vi "QuickProfile_V2.vi"(7 "Image IN":sgl[][](array[numeric]), 11 "Pixel Size (nm)":dbl, 13 "Test Image":bool) -> ()   [LabVIEW 2012]
uses:
  <vilib>/Utility/file.llb/Write To Spreadsheet File (DBL).vi
panel:
  in  "Open Image":bool
  in  "Save ROI":bool
  in  "Power (%)":dbl
  in  "Delay (ps)":dbl
  out "Lorentzian Fit Width (nm)":dbl
  out "Gaussian Fit Width Y (nm)":dbl
  out "Gaussian Fit Width X (nm)":dbl
  in  "Auto Save":bool
  in  "Save Data":bool
  in  "Save File":path
  out "Constant Y Slice":cluster{"X Values":dbl[], sgl[]}[](graph)
  out "Constant X Slice":cluster{"X Values":dbl[], sgl[]}[](graph)
  in  "Fit ROI":bool
  out "Gaussian Fit":dbl[][](graph)
  out "Lorentzian Fit":dbl[][](graph)
  out "Current ROI":sgl[][](graph)
  in  "Region Size (px)":dbl=60.0
  in  "Quit":bool
  out "Image Display":sgl[][](graph)
  # "Constant Y"
  # "Constant X"
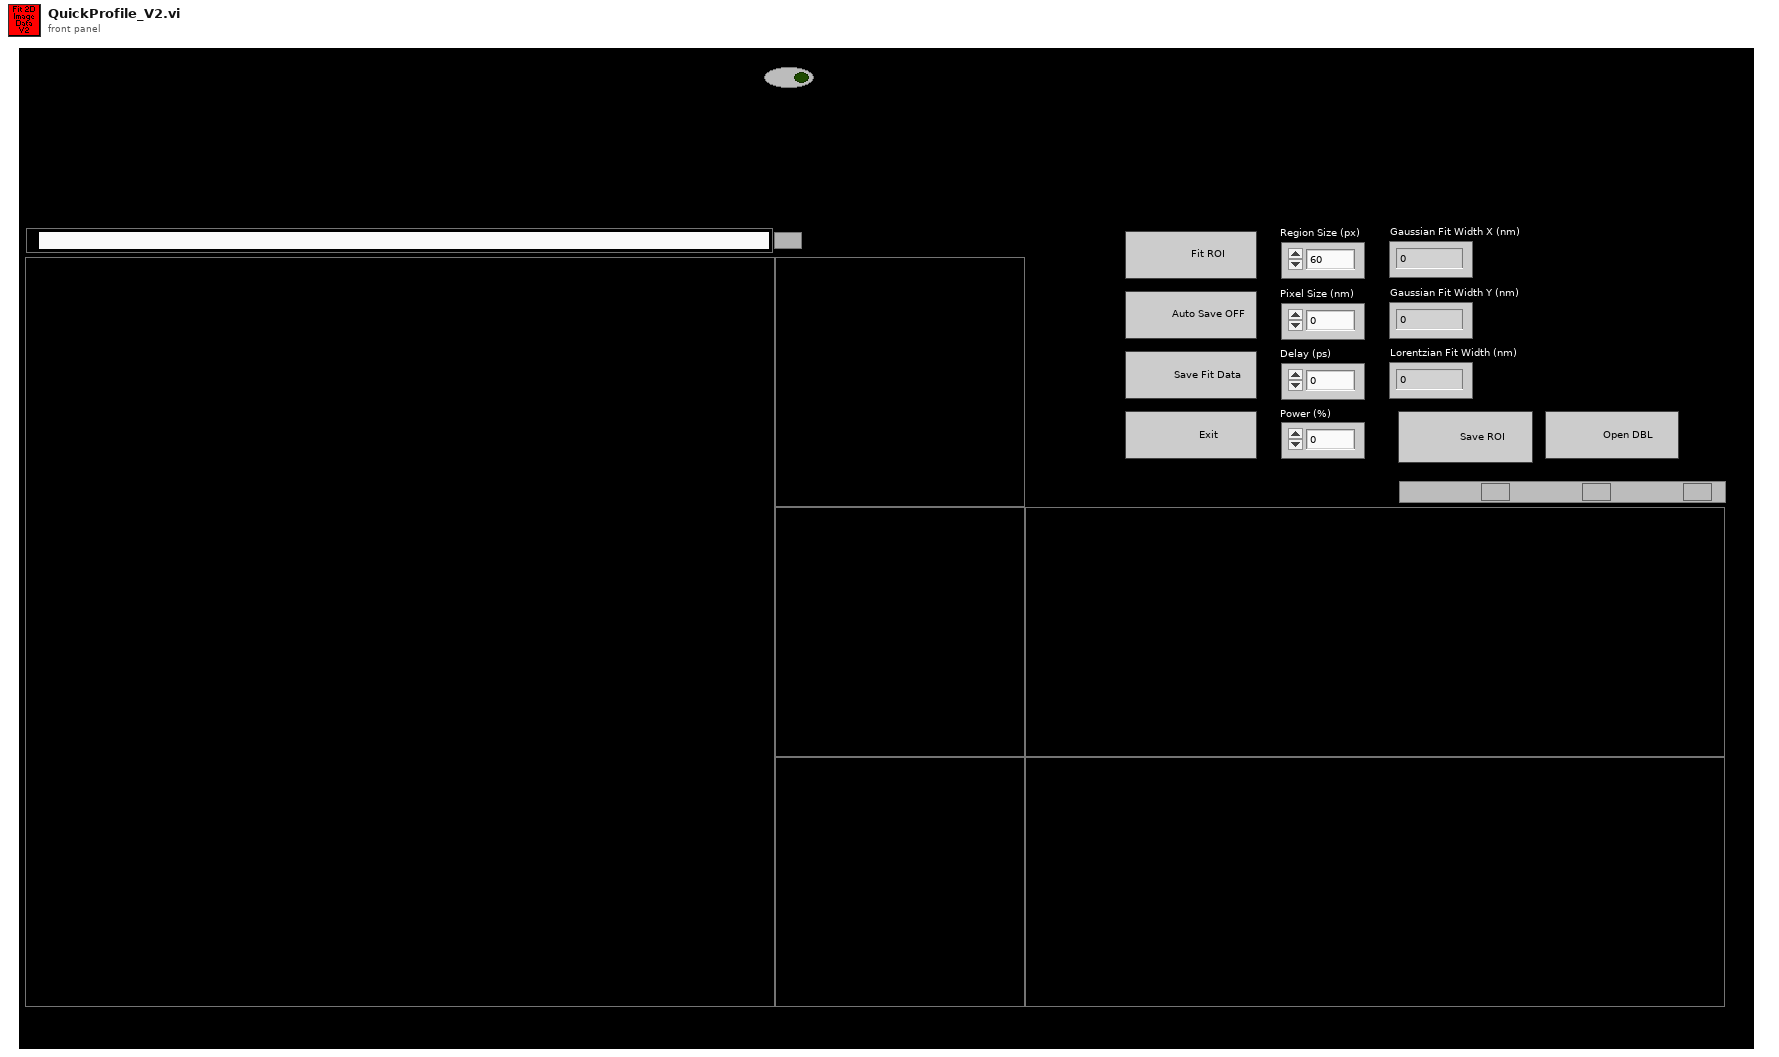
[diagram p1: front panel]
types:
  T1 = enum16{"open", "replace", "create", "open or create", "replace or create", "replace or create with confirmation"}
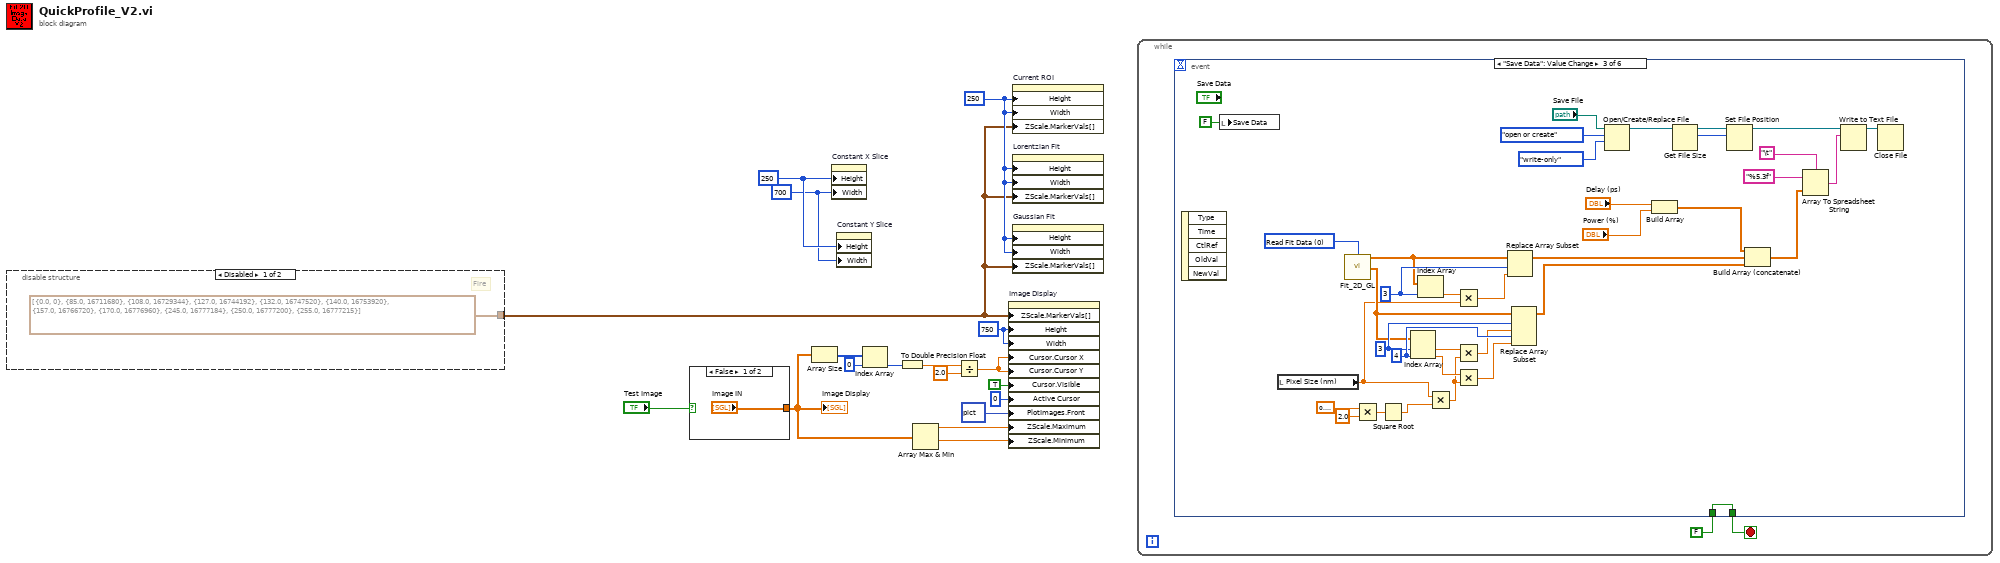
[diagram p0: block diagram]
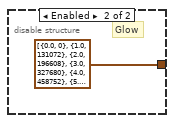
[diagram p2: hidden frame]
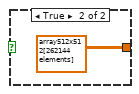
[diagram p3: hidden frame]
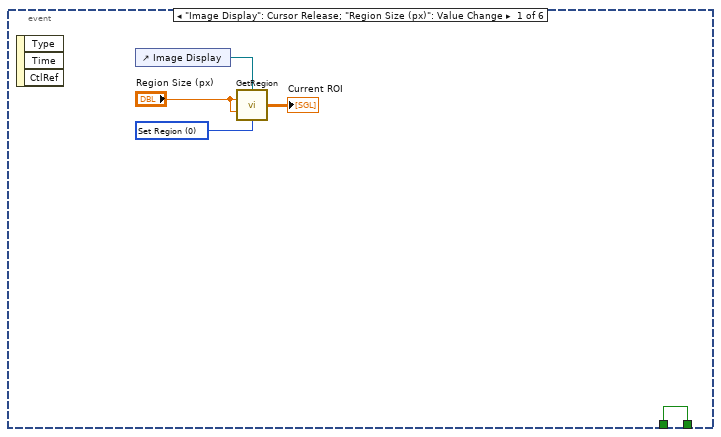
[diagram p4: hidden frame]
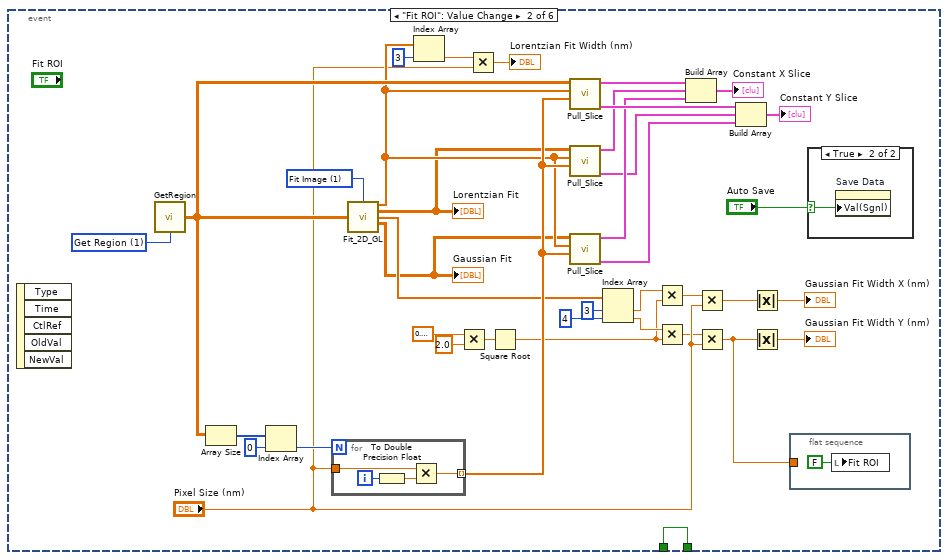
[diagram p5: hidden frame]
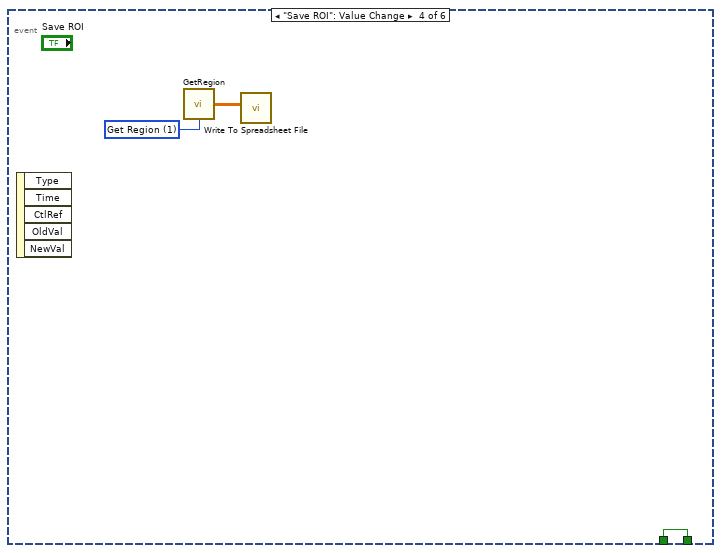
[diagram p7: hidden frame]
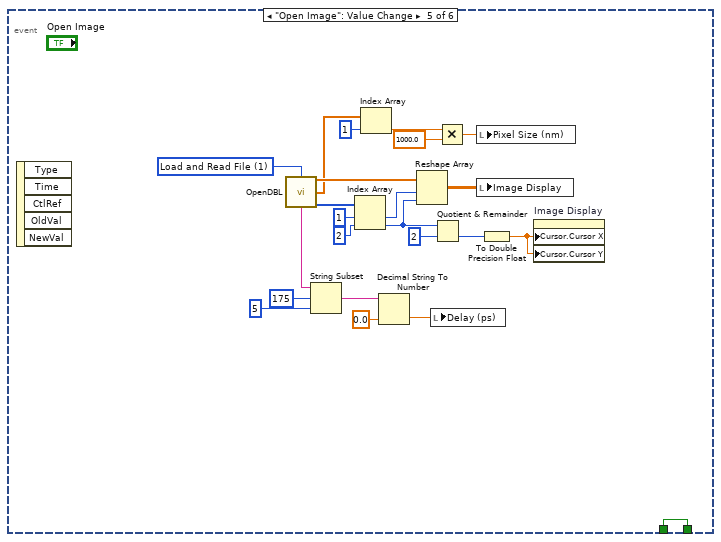
[diagram p8: hidden frame]
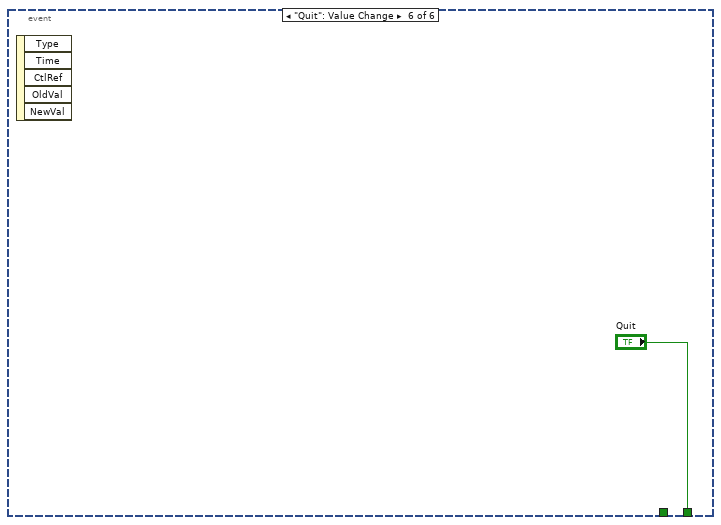
[diagram p9: hidden frame]
diagram:
  w11 = u32 700 ("Plot Area:Size:Width")
  w12 = u32 250 ("Plot Area:Size:Height")
  w14 = u32 250 ("Plot Area:Size:Height")
  w18 = u32 750 ("Plot Area:Size:Height")
  n1 = disable-structure shown="Disabled" {
    disable-tunnel: [cluster{dbl, u32}[] [{0.0, 0}, {85.0, 16711680}, {108.0, 16729344}, {127.0, 16744192}, {132.0, 16747520}, {140.0, 16753920}, {157.0, 16766720}, {170.0, 16776960}, {245.0, 16777184}, {250.0, 16777200}, {255.0, 16777215}] ("Z Scale.Marker Values[]") cluster{dbl, u32}[] [{0.0, 0}, {1.0, 131072}, {2.0, 196608}, {3.0, 327680}, {4.0, 458752}, {5.0, 589824}, {6.0, 720896}, {7.0, 851971}, {8.0, 983043}, {9.0, 1114115}, {10.0, 1245187}, {11.0, 1376259}, {12.0, 1507331}, {13.0, 1638403}, {14.0, 1769475}, {15.0, 1769479}, {16.0, 2031623}, {17.0, 2162695}, {18.0, 2293767}, {19.0, 2424839}, {20.0, 2555911}, {21.0, 2686983}, {22.0, 2818055}, {23.0, 2949127}, {24.0, 3080203}, {25.0, 3211275}, {26.0, 3342347}, {27.0, 3473419}, {28.0, 3604491}, {29.0, 3735563}, {30.0, 3866635}, {31.0, 3867403}, {32.0, 4129547}, {33.0, 4260619}, {34.0, 4391691}, {35.0, 4522763}, {36.0, 4653839}, {37.0, 4784911}, {38.0, 4915983}, {39.0, 5178127}, {40.0, 5309199}, {41.0, 5440271}, {42.0, 5571343}, {43.0, 5702415}, {44.0, 5703439}, {45.0, 5965583}, {46.0, 6096655}, {47.0, 6227727}, {48.0, 6358799}, {49.0, 6489871}, {50.0, 6620943}, {51.0, 6752015}, {52.0, 6883087}, {53.0, 7015183}, {54.0, 7146255}, {55.0, 7277327}, {56.0, 7408399}, {57.0, 7539471}, {58.0, 7670543}, {59.0, 7801615}, {60.0, 8063759}, {61.0, 8194831}, {62.0, 8326927}, {63.0, 8457999}, {64.0, 8589075}, {65.0, 8720147}, {66.0, 8851219}, {67.0, 8982291}, {68.0, 9113363}, {69.0, 9114387}, {70.0, 9376531}, {71.0, 9507603}, {72.0, 9638675}, {73.0, 9769747}, {74.0, 9901843}, {75.0, 10032915}, {76.0, 10163987}, {77.0, 10229523}, {78.0, 10295059}, {79.0, 10427155}, {80.0, 10558227}, {81.0, 10689299}, {82.0, 10820371}, {83.0, 10886931}, {84.0, 10952467}, {85.0, 11083539}, {86.0, 11214611}, {87.0, 11215635}, {88.0, 11477779}, {89.0, 11543315}, {90.0, 11608851}, {91.0, 11740947}, {92.0, 11806483}, {93.0, 11872019}, {94.0, 12004115}, {95.0, 12135187}, {96.0, 12266259}, {97.0, 12267283}, {98.0, 12398355}, {99.0, 12529427}, {100.0, 12530451}, {101.0, 12595987}, {102.0, 12530451}, {103.0, 12793619}, {104.0, 12794131}, {105.0, 12794643}, {106.0, 13056787}, {107.0, 13057299}, {108.0, 13057811}, {109.0, 13188883}, {110.0, 13320979}, {111.0, 13386515}, {112.0, 13452563}, {113.0, 13584147}, {114.0, 13584659}, {115.0, 13585171}, {116.0, 13585683}, {117.0, 13717267}, {118.0, 13848339}, {119.0, 13849363}, {120.0, 13849875}, {121.0, 13850387}, {122.0, 13981459}, {123.0, 14113555}, {124.0, 14114067}, {125.0, 14114579}, {126.0, 14115091}, {127.0, 14246675}, {128.0, 14377747}, {129.0, 14378771}, {130.0, 14379283}, {131.0, 14379539}, {132.0, 14379795}, {133.0, 14380819}, {134.0, 14511891}, {135.0, 14643987}, {136.0, 14644503}, {137.0, 14645015}, {138.0, 14645527}, {139.0, 14646039}, {140.0, 14646551}, {141.0, 14778135}, {142.0, 14909207}, {143.0, 14910231}, {144.0, 14910747}, {145.0, 14911259}, {146.0, 14911771}, {147.0, 14912283}, {148.0, 14912797}, {149.0, 15044383}, {150.0, 15175455}, {151.0, 15175967}, {152.0, 15176479}, {153.0, 15176991}, {154.0, 15177507}, {155.0, 15178019}, {156.0, 15178531}, {157.0, 15310115}, {158.0, 15441701}, {159.0, 15441959}, {160.0, 15442215}, {161.0, 15442727}, {162.0, 15443243}, {163.0, 15443755}, {164.0, 15444269}, {165.0, 15444783}, {166.0, 15444783}, {167.0, 15576367}, {168.0, 15707953}, {169.0, 15708467}, {170.0, 15708979}, {171.0, 15708981}, {172.0, 15708983}, {173.0, 15710011}, {174.0, 15710523}, {175.0, 15711037}, {176.0, 15711039}, {177.0, 15711553}, {178.0, 15843139}, {179.0, 15974213}, {180.0, 15974215}, {181.0, 15974217}, {182.0, 15974219}, {183.0, 15975755}, {184.0, 15976271}, {185.0, 15976785}, {186.0, 15977299}, {187.0, 15977301}, {188.0, 15977815}, {189.0, 15978327}, {190.0, 15978331}, {191.0, 16109917}, {192.0, 16241503}, {193.0, 16241505}, {194.0, 16242019}, {195.0, 16242535}, {196.0, 16242537}, {197.0, 16242539}, {198.0, 16243563}, {199.0, 16243567}, {200.0, 16244081}, {201.0, 16244595}, {202.0, 16244599}, {203.0, 16244601}, {204.0, 16244603}, {205.0, 16245627}, {206.0, 16245631}, {207.0, 16245633}, {208.0, 16246147}, {209.0, 16246663}, {210.0, 16377735}, {211.0, 16508811}, {212.0, 16508815}, {213.0, 16509839}, {214.0, 16509843}, {215.0, 16509845}, {216.0, 16509847}, {217.0, 16510361}, {218.0, 16510875}, {219.0, 16510879}, {220.0, 16510881}, {221.0, 16510883}, {222.0, 16511399}, {223.0, 16511911}, {224.0, 16511915}, {225.0, 16511917}, {226.0, 16511919}, {227.0, 16511923}, {228.0, 16512437}, {229.0, 16512951}, {230.0, 16512955}, {231.0, 16512957}, {232.0, 16512959}, {233.0, 16512961}, {234.0, 16512963}, {235.0, 16512967}, {236.0, 16513481}, {237.0, 16513995}, {238.0, 16513999}, {239.0, 16514001}, {240.0, 16514003}, {241.0, 16514005}, {242.0, 16514007}, {243.0, 16514011}, {244.0, 16514013}, {245.0, 16514015}, {246.0, 16514019}, {247.0, 16514021}, {248.0, 16514023}, {249.0, 16514027}, {250.0, 16514029}, {251.0, 16514031}, {252.0, 16514035}, {253.0, 16514037}, {254.0, 16514039}, {255.0, 16514043}] ("Z Scale.Marker Values[]")] -> w13
    frame Disabled {
      # "Fire"
    }
    frame Enabled {
      # "Glow"
    }
  }
  n2 = case shown="False" "Test Image" {
    tunnel: ["Image IN" sgl[][] array512x512[262144 elements] ("Im Prev")] -> w7
    frame False {
    }
    frame True {
    }
  }
  "Image Display" <- w7
  n3 = Array Size(array=w7) -> (size(s)=w6:i32[])
  n4 = property on="Constant X Slice" class="XYGraph (strict)"("Height"=w12, "Width"=w11) -> ()  [unwired: 2 in, 2 out]
  n5 = property on="Constant Y Slice" class="XYGraph (strict)"("Height"=w12, "Width"=w11) -> ()  [unwired: 2 in, 2 out]
  n6 = Index Array(array=w6, index=0) -> (element=w4:i32)
  n7 = To Double Precision Float(number=w4) -> (double precision float=w2:dbl)
  n8 = Array Max & Min(array=w7) -> (max value=w10:sgl, min value=w9:sgl)  [unwired: 2 out]
  n9 = Divide(x=w2, y=2.0) -> (x/y=w1:dbl)
  n10 = property on="Image Display" class="IntGraph (strict)"("ZScale.MarkerVals[]"=w13, "Height"=w18, "Width"=w18, "Cursor.Cursor X"=w1, "Cursor.Cursor Y"=w1, "Cursor.Visible"=TRUE, "Active Cursor"=u32 0, "PlotImages.Front"=picture data[5B] ("Plot Images:Front"), "ZScale.Maximum"=w10, "ZScale.Minimum"=w9) -> ()  [unwired: 2 in, 2 out]
  n11 = property on="Current ROI" class="IntGraph (strict)"("Height"=w14, "Width"=w14, "ZScale.MarkerVals[]"=w13) -> ()  [unwired: 2 in, 2 out]
  n12 = property on="Lorentzian Fit" class="IntGraph (strict)"("Height"=w14, "Width"=w14, "ZScale.MarkerVals[]"=w13) -> ()  [unwired: 2 in, 2 out]
  n13 = property on="Gaussian Fit" class="IntGraph (strict)"("Height"=w14, "Width"=w14, "ZScale.MarkerVals[]"=w13) -> ()  [unwired: 2 in, 2 out]
  n14 = while {
    stop <- w24 stop-if-true
    n15 = event shown="[2] \"Save Data\": Value Change" {
      selector: _ -> [_ _ _ _ _ _]
      dyn-events: _ -> [_ _ _ _ _ _]
      timeout: _ -> [_ _ _ _ _ _]
      tunnel: [w28 w68 w107 w113 w137 "Quit"] -> w24
      tunnel: FALSE -> [w28 w68 w107 w113 w137 _]
      event "Image Display": Cursor Release; "Region Size (px)": Value Change {
        w26 = u16 0 items=["Set Region", "Get Region"] ("Action")
        n16 = event-data() -> ()  [unwired: 1 in, 3 out]
        n17 = control-ref of="Image Display"() -> (w29:refnum<vi>)
        n18 = call "GetRegion.vi"("IntGraph REF"=w29, "Y Width (PX)"="Region Size (px)", "X Width (PX)"="Region Size (px)", "Action"=w26) -> ("Region Out"=→"Current ROI":sgl[][])  [unwired: 11 in]
      }
      event "Fit ROI": Value Change {
        w66 = u16 1 items=["Read Fit Data", "Fit Image"] ("Action")
        w67 = u16 1 items=["Set Region", "Get Region"] ("Action")
        n19 = event-data() -> ()  [unwired: 1 in, 5 out]
        n20 = call "GetRegion.vi"("Action"=w67) -> ("Region Out"=w56:sgl[][])  [unwired: 14 in]
        n21 = Array Size(array=w56) -> (size(s)=w65:i32[])
        n22 = Index Array(array=w65, index=0) -> (element=w63:i32)
        n23 = for {
          N: w63 -> [_]
          tunnel: "Pixel Size (nm)" -> [w73]
          tunnel: [w71] -> w62 mode=indexing
          i -> [w74]
          n24 = To Double Precision Float(number=w74) -> (double precision float=w72:dbl)
          n25 = Multiply(x=w73, y=w72) -> (x*y=w71:dbl)
        }
        n26 = call "Fit_2D_GL.vi"("Action"=w66, "Image IN"=w56) -> ("Lorentz Fit Parameters"=w51:dbl[], "Lorentzian Image"=w41:dbl[][], "Gaussian Fit Parameters"=w53:dbl[], "Gaussian Image"=w40:dbl[][])  [unwired: 10 in]
        "Gaussian Fit" <- w40
        "Lorentzian Fit" <- w41
        n27 = Index Array(array=w51, index=3) -> (element=w46:dbl)
        n28 = Multiply(x=0.6931471805599453, y=2.0) -> (x*y=w35:dbl)
        n29 = Multiply(x=w46, y="Pixel Size (nm)") -> (x*y=→"Lorentzian Fit Width (nm)":dbl)
        n30 = Square Root(x=w35) -> (sqrt(x)=w32:dbl)
        n31 = call "Pull_Slice.vi"("X Values"=w62, "Fit Parameters"=w51, "ROI Image"=w56) -> ("Constant X Slice"=w61:cluster{"X Values":dbl[], sgl[]}, "Constant Y Slice"=w47:cluster{"X Values":dbl[], sgl[]})  [unwired: 7 in]
        n32 = call "Pull_Slice.vi"("X Values"=w62, "Fit Parameters"=w51, "ROI Image"=w41) -> ("Constant X Slice"=w58:cluster{"X Values":dbl[], sgl[]}, "Constant Y Slice"=w60:cluster{"X Values":dbl[], sgl[]})  [unwired: 7 in]
        n33 = call "Pull_Slice.vi"("X Values"=w62, "Fit Parameters"=w51, "ROI Image"=w40) -> ("Constant X Slice"=w57:cluster{"X Values":dbl[], sgl[]}, "Constant Y Slice"=w59:cluster{"X Values":dbl[], sgl[]})  [unwired: 7 in]
        n34 = Index Array(array=w53, index #1=3 ("index"), index #2=4 ("index")) -> (element #1=w39:dbl, element #2=w37:dbl)
        n35 = Multiply(x=w39, y=w32) -> (x*y=w38:dbl)
        n36 = Multiply(x=w37, y=w32) -> (x*y=w36:dbl)
        n37 = Build Array(w47, w60, w59) -> (→"Constant X Slice":cluster{"X Values":dbl[], sgl[]}[])
        n38 = Multiply(x=w38, y="Pixel Size (nm)") -> (x*y=w44:dbl)
        n39 = Multiply(x=w36, y="Pixel Size (nm)") -> (x*y=w42:dbl)
        n40 = Build Array(w61, w58, w57) -> (→"Constant Y Slice":cluster{"X Values":dbl[], sgl[]}[])
        n41 = Absolute Value(x=w44) -> (abs(x)=→"Gaussian Fit Width X (nm)":dbl)
        n42 = Absolute Value(x=w42) -> (abs(x)=→"Gaussian Fit Width Y (nm)":dbl)
        n43 = flat-sequence {
          tunnel: w42 -> [_]
          frame #0 {
            n44 = local write "Fit ROI"(FALSE ("Fit ROI")) -> ()
          }
        }
        n45 = case shown="True" "Auto Save" {
          selector: "Auto Save" -> [_ w70]
          frame False {
          }
          frame True {
            n46 = property on="Save Data" class="Bool (strict)"("Val(Sgnl)"=w70) -> ()  [unwired: 2 in, 2 out]
          }
        }
      }
      event "Save Data": Value Change {
        w94 = 4 ("index")
        w93 = 3 ("index")
        w85 = 3 ("index")
        w83 = u16 0 items=["Read Fit Data", "Fit Image"] ("Action")
        n47 = event-data() -> ()  [unwired: 1 in, 5 out]
        n48 = local write "Save Data"(FALSE ("Save Data")) -> ()
        n49 = local read "Pixel Size (nm)"() -> (w75:dbl)
        n50 = call "Fit_2D_GL.vi"("Action"=w83) -> ("Lorentz Fit Parameters"=w84:dbl[], "Gaussian Fit Parameters"=w88:dbl[])  [unwired: 11 in, 2 out]
        n51 = Multiply(x=0.6931471805599453, y=2.0) -> (x*y=w80:dbl)
        n52 = Square Root(x=w80) -> (sqrt(x)=w77:dbl)
        n53 = Index Array(array=w88, index #1=w93, index #2=w94) -> (element #1=w89:dbl, element #2=w90:dbl)
        n54 = Index Array(array=w84, index=w85) -> (element=w86:dbl)
        n55 = Multiply(x=w75, y=w77) -> (x*y=w76:dbl)
        n56 = Multiply(x=w86, y=w75) -> (x*y=w87:dbl)
        n57 = Multiply(x=w89, y=w76) -> (x*y=w91:dbl)
        n58 = Multiply(x=w90, y=w76) -> (x*y=w92:dbl)
        n59 = Replace Array Subset(array=w84, new element=w87, index=w85) -> (w82:dbl[])
        n60 = Replace Array Subset(array=w88, new element #1=w91, index #1=w93, new element #2=w92, index #2=w94) -> (w81:dbl[])
        n61 = Open/Create/Replace File(file path (use dialog)="Save File", operation (0:open)=T1."open or create", access (0:read/write)=enum16{"read/write", "read-only", "write-only"}."write-only") -> (refnum out=w104:refnum<file>)  [unwired: 3 in, 2 out]
        n62 = Build Array("Delay (ps)", "Power (%)") -> (w95:dbl[])
        n63 = Get File Size(file=w104) -> (refnum out=w103:refnum<file>, size (in bytes)=w105:i64)  [unwired: 1 in, 1 out]
        n64 = Set File Position(offset (in bytes) (0)=w105, refnum=w103) -> (refnum out=w106:refnum<file>)  [unwired: 2 in, 1 out]
        n65 = Build Array (concatenate)(w95, w82, w81) -> (w98:dbl[])
        n66 = Array To Spreadsheet String(delimiter (Tab)="\t", array=w98, 3:"%5.3f" ("format string")) -> (spreadsheet string=w100:string)
        n67 = Write to Text File(file (use dialog)=w106, text=w100) -> (refnum out=w108:refnum<file>)  [unwired: 2 in, 2 out]
        n68 = Close File(refnum=w108) -> ()  [unwired: 1 in, 2 out]
      }
      event "Save ROI": Value Change {
        w114 = u16 1 items=["Set Region", "Get Region"] ("Action")
        n69 = event-data() -> ()  [unwired: 1 in, 5 out]
        n70 = call "GetRegion.vi"("Action"=w114) -> ("Region Out"=w112:sgl[][])  [unwired: 14 in]
        n71 = call-poly <vilib>:"Write To Spreadsheet File.vi"("2D data"=w112) -> ()  [unwired: 7 in, 1 out]
      }
      event "Open Image": Value Change {
        w136 = u16 1 items=["Get Image", "Load and Read File"] ("Action")
        n72 = event-data() -> ()  [unwired: 1 in, 5 out]
        n73 = call "OpenDBL.vi"("Action"=w136) -> ("Image"=w135:sgl[], "Physical Length (Z, Y, X, t)"=w129:sgl[], "File Notes"=w120:string, "Dimensions (Z, Y, X, t)"=w134:i32[])  [unwired: 11 in]
        n74 = String Subset(string=w120, offset (0)=175, length (rest)=5 ("length (rest)")) -> (substring=w117:string)
        n75 = Index Array(array=w134, index #1=1 ("index"), index #2=2 ("index")) -> (element #1=w131:i32, element #2=w124:i32)
        n76 = Index Array(array=w129, index=1) -> (element=w127:sgl)
        n77 = Decimal String To Number(string=w117, default (0L)=0.0 ("default (0 I32)")) -> (number=w115:dbl)  [unwired: 1 in, 1 out]
        n78 = Reshape Array(w135, w131, w124) -> (w130:sgl[][])
        n79 = local write "Delay (ps)"(w115) -> ()
        n80 = Quotient & Remainder(x=w124, y=2) -> (floor(x/y)=w122:i32)  [unwired: 1 out]
        n81 = Multiply(x=w127, y=sgl 1000.0) -> (x*y=w125:sgl)
        n82 = local write "Pixel Size (nm)"(w125) -> ()
        n83 = local write "Image Display"(w130) -> ()
        n84 = To Double Precision Float(number=w122) -> (double precision float=w121:dbl)
        n85 = property on="Image Display" class="IntGraph (strict)"("Cursor.Cursor X"=w121, "Cursor.Cursor Y"=w121) -> ()  [unwired: 2 in, 2 out]
      }
      event "Quit": Value Change {
        n86 = event-data() -> ()  [unwired: 1 in, 5 out]
      }
    }
  }
